vi "SetMultipleChannelValues.vi"(8 "error in (no error)":errorcluster, 10 "Channel Key Value Pairs in":T1[](array[typedef]), 11 "VeriStandTestCase in":refnum<class "VeriStandTestCase.lvclass">) -> (0 "error out":errorcluster, 3 "VeriStandTestCase out":refnum<class "VeriStandTestCase.lvclass">)   [LabVIEW 2027, in "VeriStandTestCase.lvclass"]
uses:
  VeriStandTestCase.lvclass
  Utilities/ChannelKeyValuePair.ctl
  <vilib>/NI VeriStand/Execution/Workspace/NI VeriStand - Set Multiple Channel Values.vi
  <vilib>/NI VeriStand/Execution/Workspace/NI_VS Workspace ExecutionAPI.lvlib
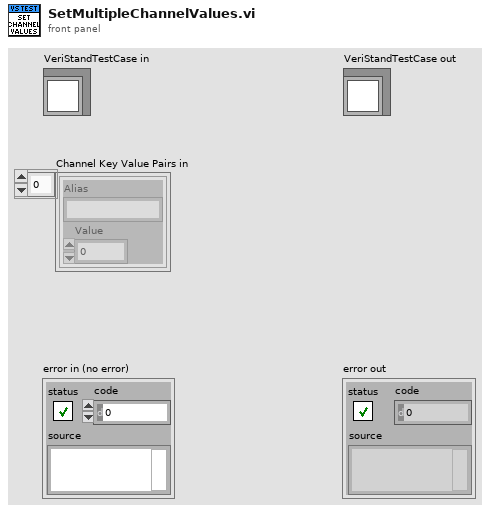
[diagram p1: front panel]
types:
  T1 = typedef "VeriStandTestCase.lvclass/ChannelKeyValuePair.ctl" = cluster{"Alias":string, "Value":dbl}
  T2 = typedef "NI_VS Workspace ExecutionAPI.lvlib/WorkspaceAPI.ctl" = refnum<k39>
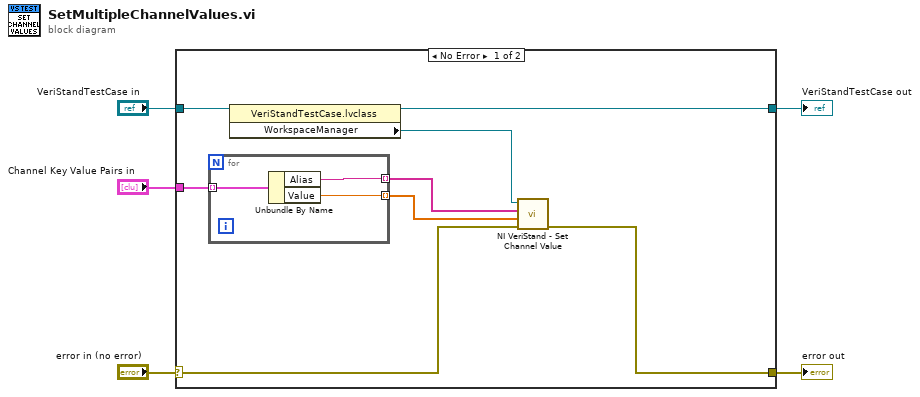
[diagram p0: block diagram]
diagram:
  n1 = case shown="No Error" "error in (no error)" {
    selector: "error in (no error)" -> [w13 w18]
    tunnel: [w12 w18] -> w2
    tunnel: [w10 w17] -> w4
    tunnel: "VeriStandTestCase in" -> [w11 w17]
    tunnel: "Channel Key Value Pairs in" -> [w9 _]
    frame No Error {
      n2 = for {
        tunnel: [w16] -> w7 mode=indexing
        tunnel: [w15] -> w6 mode=indexing
        tunnel: w9 -> [w14] mode=indexing
        n3 = Unbundle By Name(w14) -> ("Alias"=w16:string, "Value"=w15:dbl)
      }
      n4 = property class="VeriStandTestCase.lvclass"(reference=w11) -> (reference out=w10:refnum<class "VeriStandTestCase.lvclass">, "WorkspaceManager"=w8:T2)  [unwired: 1 in, 1 out]
      n5 = call-poly <vilib>:"NI VeriStand - Set Channel Value.vi"("error in (no error)"=w13, "Values"=w6, "Channels"=w7, "WorkspaceManager in"=w8) -> ("error out"=w12:errorcluster)  [unwired: 6 in, 1 out]
    }
    frame Error {
    }
  }
  "error out" <- w2
  "VeriStandTestCase out" <- w4
